vi "_keysight_setup.vi"(0 "Frequency Parameters":T2={"Coupling"=FALSE, "Frequency 2 (MHz)"=1.0, "Frequency 1 (MHz)"=1.0, "WAVEFORM"=enum."PULSE"} {"Frequency 1 (MHz)" min=0.0 max=14.5; "Frequency 2 (MHz)" min=0.0 max=14.5}, 1 "Outputs":T3={"Ouput 1"=TRUE, "Ouput 2"=TRUE, "Ouput 1 Neg"=TRUE, "Ouput 2 Neg"=TRUE}, 3 "error in":errorcluster, 4 "Keysight Connection":T1={"Type"=1, "VISA"="TCPIP0::192.168.0.8::inst0::INSTR", "GPIB"="10"} {"Type" items=["VISA", "GPIB"]}) -> (6 "error out":errorcluster)   [LabVIEW 2013]
panel:
  out "Command":string=":track:channel1 ON\n:frequency1 2.000MHz\n:output1 ON\n:output2 ON\n:output1:complement ON\n:output2:complement ON\n:output1:strobe:route NONE\n:output2:strobe:route NONE\n:output1:trigger:route SYNA\n:output2:trigger:route SYNB\n:SOURCE:VOLTAGE2:HIGH 4\n:SOURCE:VOLTAGE2:LOW 0\n:SOURCE:VOLTAGE1:HIGH 4\n:SOURCE:VOLTAGE1:LOW 0"
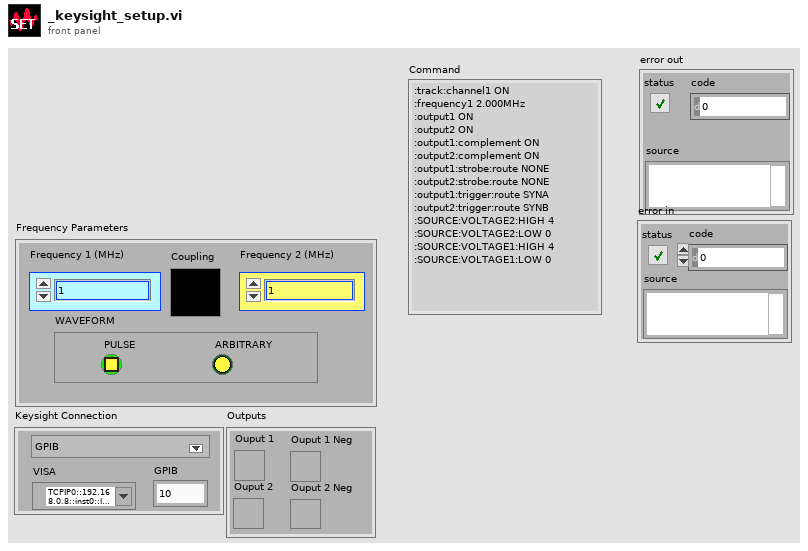
[diagram p1: front panel]
types:
  T1 = cluster{"Type":u16, "VISA":refnum<visa-resource-name>, "GPIB":string}
  T2 = cluster{"Coupling":bool, "Frequency 2 (MHz)":dbl, "Frequency 1 (MHz)":dbl, "WAVEFORM":enum32{"PULSE", "ARBITRARY"}}
  T3 = cluster{"Ouput 1":bool, "Ouput 2":bool, "Ouput 1 Neg":bool, "Ouput 2 Neg":bool}
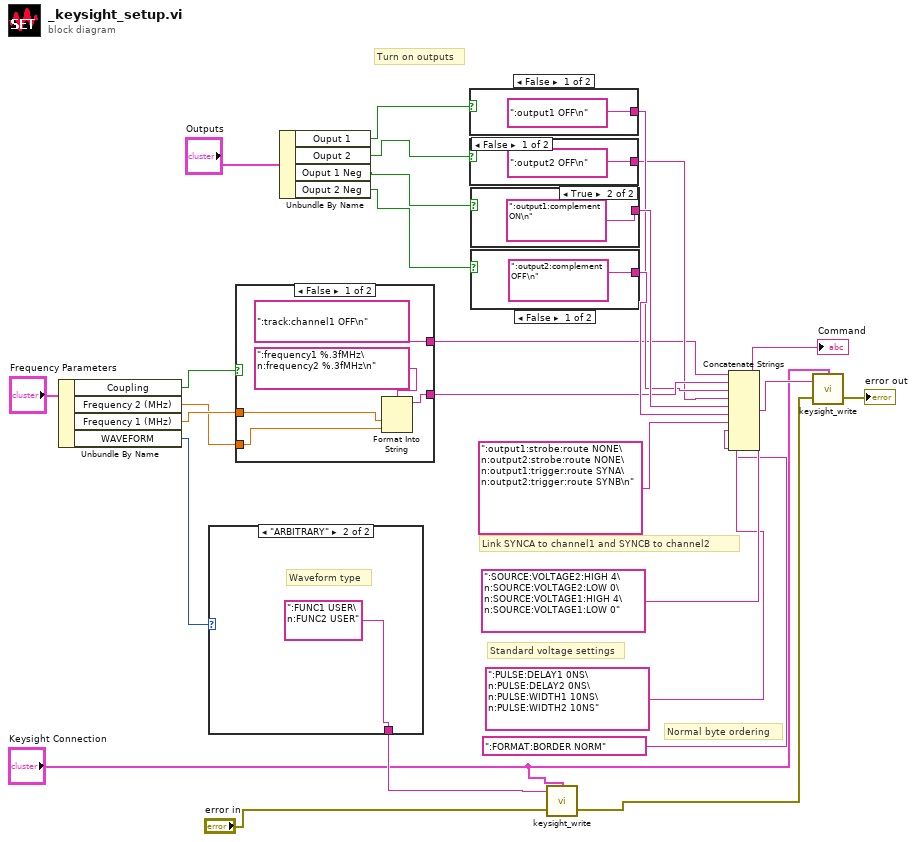
[diagram p0: block diagram]
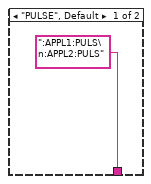
[diagram p2: hidden frame]
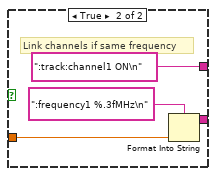
[diagram p3: hidden frame]
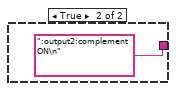
[diagram p4: hidden frame]
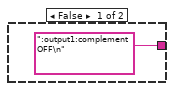
[diagram p5: hidden frame]
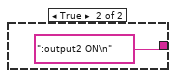
[diagram p6: hidden frame]
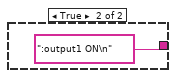
[diagram p7: hidden frame]
diagram:
  # "Normal byte ordering"
  # "Standard voltage settings"
  # "Link SYNCA to channel1 and SYNCB to channel2"
  # "Turn on outputs"
  n1 = Unbundle By Name("Frequency Parameters") -> ("Coupling"=w11:bool, "Frequency 2 (MHz)"=w9:dbl, "Frequency 1 (MHz)"=w10:dbl, "WAVEFORM"=w7:enum32{"PULSE", "ARBITRARY"})
  n2 = case shown="\"ARBITRARY\"" w7 {
    tunnel: [":APPL1:PULS\n:APPL2:PULS" ("string") ":FUNC1 USER\n:FUNC2 USER" ("string")] -> w5
    frame "PULSE", Default {
    }
    frame "ARBITRARY" {
      # "Waveform type"
    }
  }
  n3 = case shown="False" w11 {
    tunnel: w10 -> [w32 w36]
    tunnel: [w30 w35] -> w24
    tunnel: w9 -> [w31 _]
    tunnel: [":track:channel1 OFF\n" ":track:channel1 ON\n"] -> w20
    frame False {
      n4 = Format Into String(format string=":frequency1 %.3fMHz\n:frequency2 %.3fMHz\n", w32, w31) -> (resulting string=w30:string)  [unwired: 2 in, 1 out]
    }
    frame True {
      # "Link channels if same frequency"
      n5 = Format Into String(format string=":frequency1 %.3fMHz\n", w36) -> (resulting string=w35:string)  [unwired: 2 in, 1 out]
    }
  }
  n6 = Unbundle By Name("Outputs") -> ("Ouput 1"=w16:bool, "Ouput 2"=w15:bool, "Ouput 1 Neg"=w14:bool, "Ouput 2 Neg"=w13:bool)
  n7 = case shown="False" w16 {
    tunnel: [":output1 OFF\n" ":output1 ON\n"] -> w23
    frame False {
    }
    frame True {
    }
  }
  n8 = case shown="False" w15 {
    tunnel: [":output2 OFF\n" ":output2 ON\n"] -> w22
    frame False {
    }
    frame True {
    }
  }
  n9 = case shown="True" w14 {
    tunnel: [":output1:complement OFF\n" ":output1:complement ON\n"] -> w26
    frame False {
    }
    frame True {
    }
  }
  n10 = case shown="False" w13 {
    tunnel: [":output2:complement OFF\n" ":output2:complement ON\n"] -> w25
    frame False {
    }
    frame True {
    }
  }
  n11 = call "keysight_write.vi"("error in"="error in", "command"=w5, "Connection"="Keysight Connection") -> ("error out"=w4:errorcluster)  [unwired: 1 in]
  n12 = Concatenate Strings(w20, w24, w23, w22, w26, w25, ":output1:strobe:route NONE\n:output2:strobe:route NONE\n:output1:trigger:route SYNA\n:output2:trigger:route SYNB\n", ":SOURCE:VOLTAGE2:HIGH 4\n:SOURCE:VOLTAGE2:LOW 0\n:SOURCE:VOLTAGE1:HIGH 4\n:SOURCE:VOLTAGE1:LOW 0", ":PULSE:DELAY1 0NS\n:PULSE:DELAY2 0NS\n:PULSE:WIDTH1 10NS\n:PULSE:WIDTH2 10NS", ":FORMAT:BORDER NORM") -> (w19:string)
  "Command" <- w19
  n13 = call "keysight_write.vi"("error in"=w4, "command"=w19, "Connection"="Keysight Connection") -> ("error out"=→"error out":errorcluster)  [unwired: 1 in]
